vi "Test - Polymorphic.vi"   [LabVIEW 2015, in "ByRef Variant Repository.lvlib"]
uses:
  ByRef Variant Repository.lvlib
  Get (Boolean Array).vi
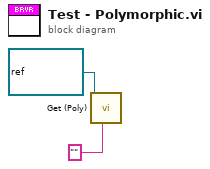
[diagram p0: block diagram]
diagram:
  n1 = call-poly "Get (Poly).vi"("Tag"="", "ByRef Variant Repsitory in"=refnum<data-value> refnum) -> ()  [unwired: 7 in, 2 out]
